vi "Acquire-b.vi"() -> (0 "Waveform Chart":dbl(graph))   [LabVIEW 2020]
doc: "This vi is used to acquire data from a LV2"
uses:
  Typedefs/Stop cases.ctl
  Typedefs/LV2 numeric.ctl
panel:
  out "Error out":errorcluster
  in  "Error in":errorcluster
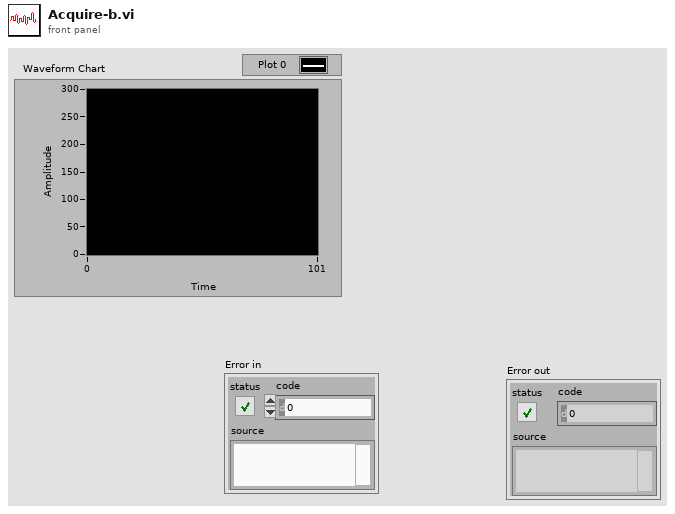
[diagram p1: front panel]
types:
  T1 = typedef "Stop cases.ctl" = enum16{"Initialize", "Write", "Read"}
  T2 = typedef "LV2 numeric.ctl" = enum16{"Initialize", "Read", "Write"}
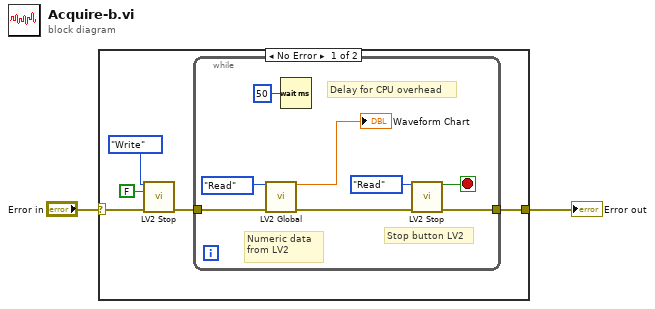
[diagram p0: block diagram]
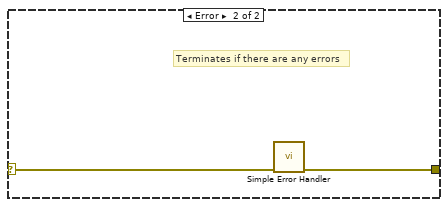
[diagram p2: hidden frame]
diagram:
  n1 = case shown="No Error" "Error in" {
    selector: "Error in" -> [w5 w16]
    tunnel: [w3 w17] -> w2
    frame No Error {
      n2 = call "LV2 Stop.vi"("Operation"=Stop_cases."Write", "Stop"=FALSE, "Error in"=w5) -> ("Error out"=w4:errorcluster)  [unwired: 11 in, 1 out]
      n3 = while {
        tunnel: w4 -> [w11]
        tunnel: [w9] -> w3
        stop <- w15 stop-if-true
        # "Stop button LV2"
        # "Numeric data \nfrom LV2"
        # "Delay for CPU overhead"
        n4 = call "LV2 Global.vi"("Operation"=LV2_numeric."Read", "Error in"=w11) -> ("Numeric Output"=→"Waveform Chart":dbl, "Error out"=w10:errorcluster)  [unwired: 12 in]
        n5 = Wait (ms)(milliseconds to wait=u32 50) -> ()  [unwired: 1 out]
        n6 = call "LV2 Stop.vi"("Operation"=Stop_cases."Read", "Error in"=w10) -> ("Output"=w15:bool, "Error out"=w9:errorcluster)  [unwired: 12 in]
      }
    }
    frame Error {
      # "Terminates if there are any errors"
      n7 = call <vilib>:"Simple Error Handler.vi"("error in (no error)"=w16) -> ("error out"=w17:errorcluster)  [unwired: 4 in, 4 out]
    }
  }
  "Error out" <- w2
